vi "Cache.StatusUpdate.vi"(7 "Idx":i32, 8 "error in (no error)":errorcluster, 11 "Data in":T1) -> (0 "error out":errorcluster, 3 "Data out":T1)   [LabVIEW 2016]
uses:
  Cache.Data.ctl
  Cache.Data.Status.ctl
  Cache.Data.Sets.ctl
  Database/Database.Global.vi
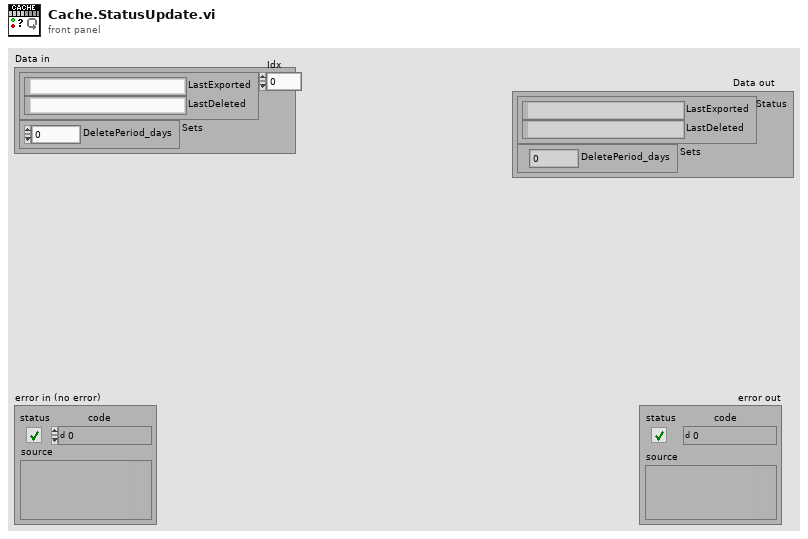
[diagram p1: front panel]
types:
  T1 = typedef "Cache.Data.ctl" = cluster{"Status":T2, "Sets":T3}
  T2 = typedef "Cache.Data.Status.ctl" = cluster{"LastExported":string, "LastDeleted":string}
  T3 = typedef "Cache.Data.Sets.ctl" = cluster{"DeletePeriod_days":dbl}
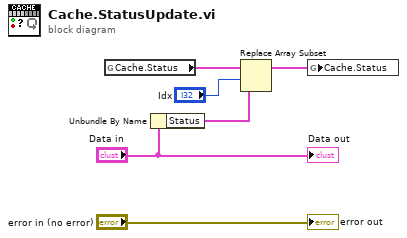
[diagram p0: block diagram]
diagram:
  n1 = global read "Database.Global.vi" "Cache.Status"() -> (w3:T2[])
  n2 = Unbundle By Name("Data in") -> ("Status"=w1:T2)
  n3 = Replace Array Subset(array=w3, new element=w1, index="Idx") -> (w2:T2[])
  n4 = global write "Database.Global.vi" "Cache.Status"(w2) -> ()
  "Data out" <- "Data in"
  "error out" <- "error in (no error)"
